vi "Handle Mouse State Change.vi"(8 "error in (no error)":errorcluster, 9 "Mouse Down":bool, 10 "Mouse Coordinates":T1, 11 "Toolbar Control in":refnum<class "Toolbar Control.lvclass">) -> (0 "error out":errorcluster, 1 "Toolbar Image":picture, 2 "Update Toolbar":bool, 3 "Toolbar Control out":refnum<class "Toolbar Control.lvclass">)   [LabVIEW 2011, in "Toolbar Control.lvclass"]
doc: "This VI handles the Mouse State Change event on the toolbar. When the Mouse Moves, or a Mouse Down is detected run this VI providing the current <B>Mouse Coordinates</B>, and if the <B>Mouse is Down</B>.\n\n-------------\nDeveloped by Brian Hoover (hooovahh)"
uses:
  Toolbar Control.lvclass
  <vilib>/Utility/miscctls.llb/LVPoint32TypeDef.ctl
  Toolbar Control.lvclass/Toolbar Control.ctl
  Controls/Mouse State.ctl
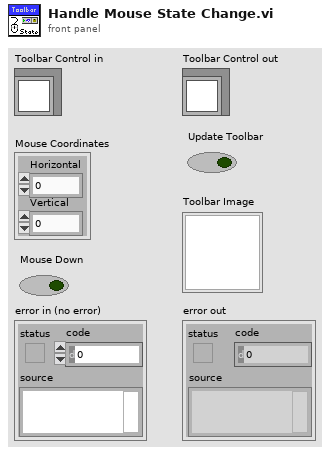
[diagram p1: front panel]
types:
  T1 = typedef "LVPoint32TypeDef.ctl" = cluster{"Horizontal":i32, "Vertical":i32}
  T2 = typedef "Mouse State.ctl" = enum8{"Normal", "Mouse Over", "Mouse Down"}
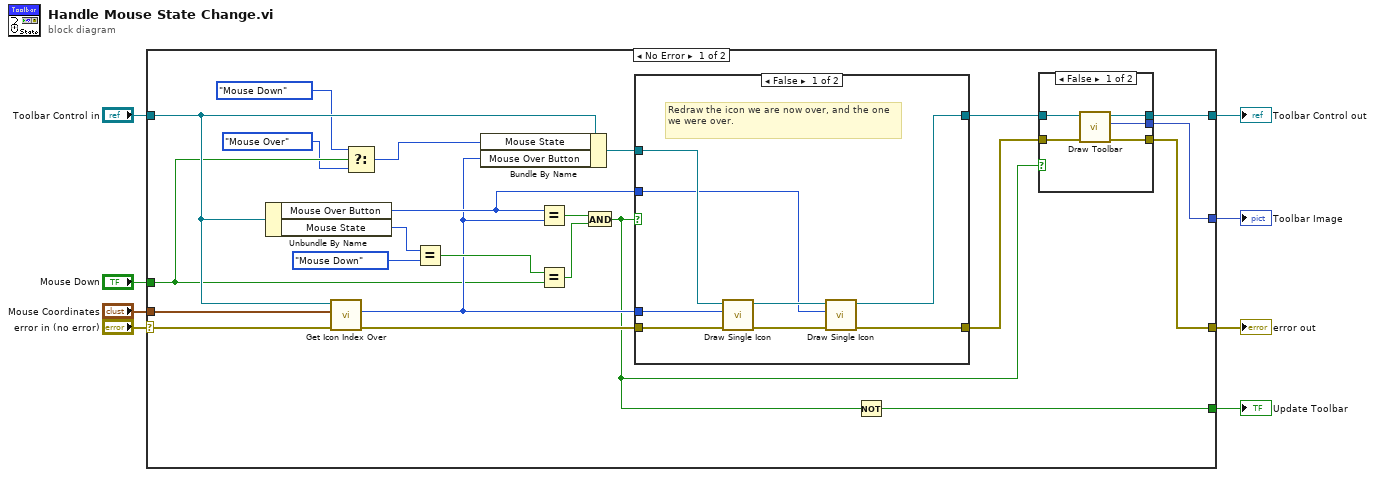
[diagram p0: block diagram]
diagram:
  n1 = case shown="No Error" "error in (no error)" {
    selector: "error in (no error)" -> [w24 w49]
    tunnel: [w20 w50] -> w6
    tunnel: "Toolbar Control in" -> [w25 w50]
    tunnel: "Mouse Coordinates" -> [w31 _]
    tunnel: "Mouse Down" -> [w13 _]
    tunnel: [w19 _] -> w3
    tunnel: [w17 w49] -> w2
    tunnel: [w22 _] -> w1
    frame No Error {
      n2 = Unbundle By Name(w25) -> ("Mouse Over Button"=w15:i32, "Mouse State"=w30:T2)
      n3 = call "Get Icon Index Over.vi"("error in (no error)"=w24, "Mouse Coordinates"=w31, "Toolbar Control in"=w25) -> ("error out"=w23:errorcluster, "Icon Index Over"=w14:i32)  [unwired: 4 in, 3 out]
      n4 = Select(t=Mouse_State."Mouse Down" ("Mouse State"), s=w13, f=Mouse_State."Mouse Over" ("Mouse State")) -> (s? t:f=w11:T2)
      n5 = Equal?(x=w30, y=Mouse_State."Mouse Down" ("Mouse State")) -> (x = y?=w28:bool)
      n6 = Bundle By Name(cluster=w25, "Mouse State"=w11, "Mouse Over Button"=w14) -> (w21:refnum<class "Toolbar Control.lvclass">)
      n7 = Equal?(x=w15, y=w14) -> (x = y?=w27:bool)
      n8 = Equal?(x=w28, y=w13) -> (x = y?=w26:bool)
      n9 = And(x=w27, y=w26) -> (x .and. y?=w9:bool)
      n10 = case shown="False" w9 {
        tunnel: w21 -> [w46 w48]
        tunnel: [w43 w48] -> w18
        tunnel: w23 -> [w45 w47]
        tunnel: [w41 w47] -> w16
        tunnel: w15 -> [w40 _]
        tunnel: w14 -> [w39 _]
        frame False {
          # "Redraw the icon we are now over, and the one we were over."
          n11 = call "Draw Single Icon.vi"("error in (no error)"=w45, "Icon Index"=w39, "Toolbar Control in"=w46) -> ("error out"=w42:errorcluster, "Toolbar Control out"=w44:refnum<class "Toolbar Control.lvclass">)  [unwired: 7 in]
          n12 = call "Draw Single Icon.vi"("error in (no error)"=w42, "Icon Index"=w40, "Toolbar Control in"=w44) -> ("error out"=w41:errorcluster, "Toolbar Control out"=w43:refnum<class "Toolbar Control.lvclass">)  [unwired: 7 in]
        }
        frame True {
          # "No change in mouse state"
        }
      }
      n13 = Not(x=w9) -> (.not. x?=w22:bool)
      n14 = case shown="False" w9 {
        tunnel: [w36 w37] -> w20
        tunnel: [w35 _] -> w19
        tunnel: w18 -> [w34 w37]
        tunnel: [w33 w38] -> w17
        tunnel: w16 -> [w32 w38]
        frame False {
          n15 = call "Draw Toolbar.vi"("error in (no error)"=w32, "Toolbar Control in"=w34) -> ("error out"=w33:errorcluster, "Toolbar Image"=w35:picture, "Toolbar Control out"=w36:refnum<class "Toolbar Control.lvclass">)  [unwired: 7 in]
        }
        frame True {
        }
      }
    }
    frame Error {
    }
  }
  "error out" <- w2
  "Toolbar Control out" <- w6
  "Toolbar Image" <- w3
  "Update Toolbar" <- w1
